vi "Periodic Tasks.vi"(0 "error in":errorcluster) -> ()   [LabVIEW 2019]
doc: "This VI runs in parallel to other tasks. It can contain as many user-defined periodic loops as you need. These can carry out PID or other sorts of timed response."
uses:
  dsinstructions.vi
  outputs.vi
  dsdata.vi
  constants.vi
  autoinfo.vi
  sensors.vi
  23a3f555-9381-40b3-b51f-cf650278d793.vi
  <vilib>/Rock Robotics/Network Tables/NT Write Number.vi
  8c2ce585-3354-44ed-b83e-22b56f2f092c.vi
  bb0a537a-131d-4120-96fe-e8b26fcd9fb4.vi
  <vilib>/Rock Robotics/Network Tables/NT Write String.vi
  70680724-1a9c-4240-8929-d59eeec2e4a0.vi
panel:
  out "Drive Sequencer":i32
  out "Subsystem Action":path
  out "Time Since Latch (ms)":u32
  out "Subsystem Sequencer":i32
  out "Drive Action":string
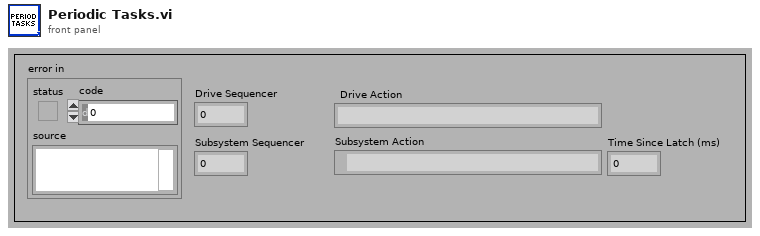
[diagram p1: front panel]
types:
  T1 = typedef "WPI_DriverStationRobotMode2.ctl" = enum16{"Autonomous Disabled", "Autonomous Enabled", "Teleop Disabled", "Teleop Enabled", "Disconnected", "Finish", "Test Disabled", "Test Enabled", "Emergency Stopped"}
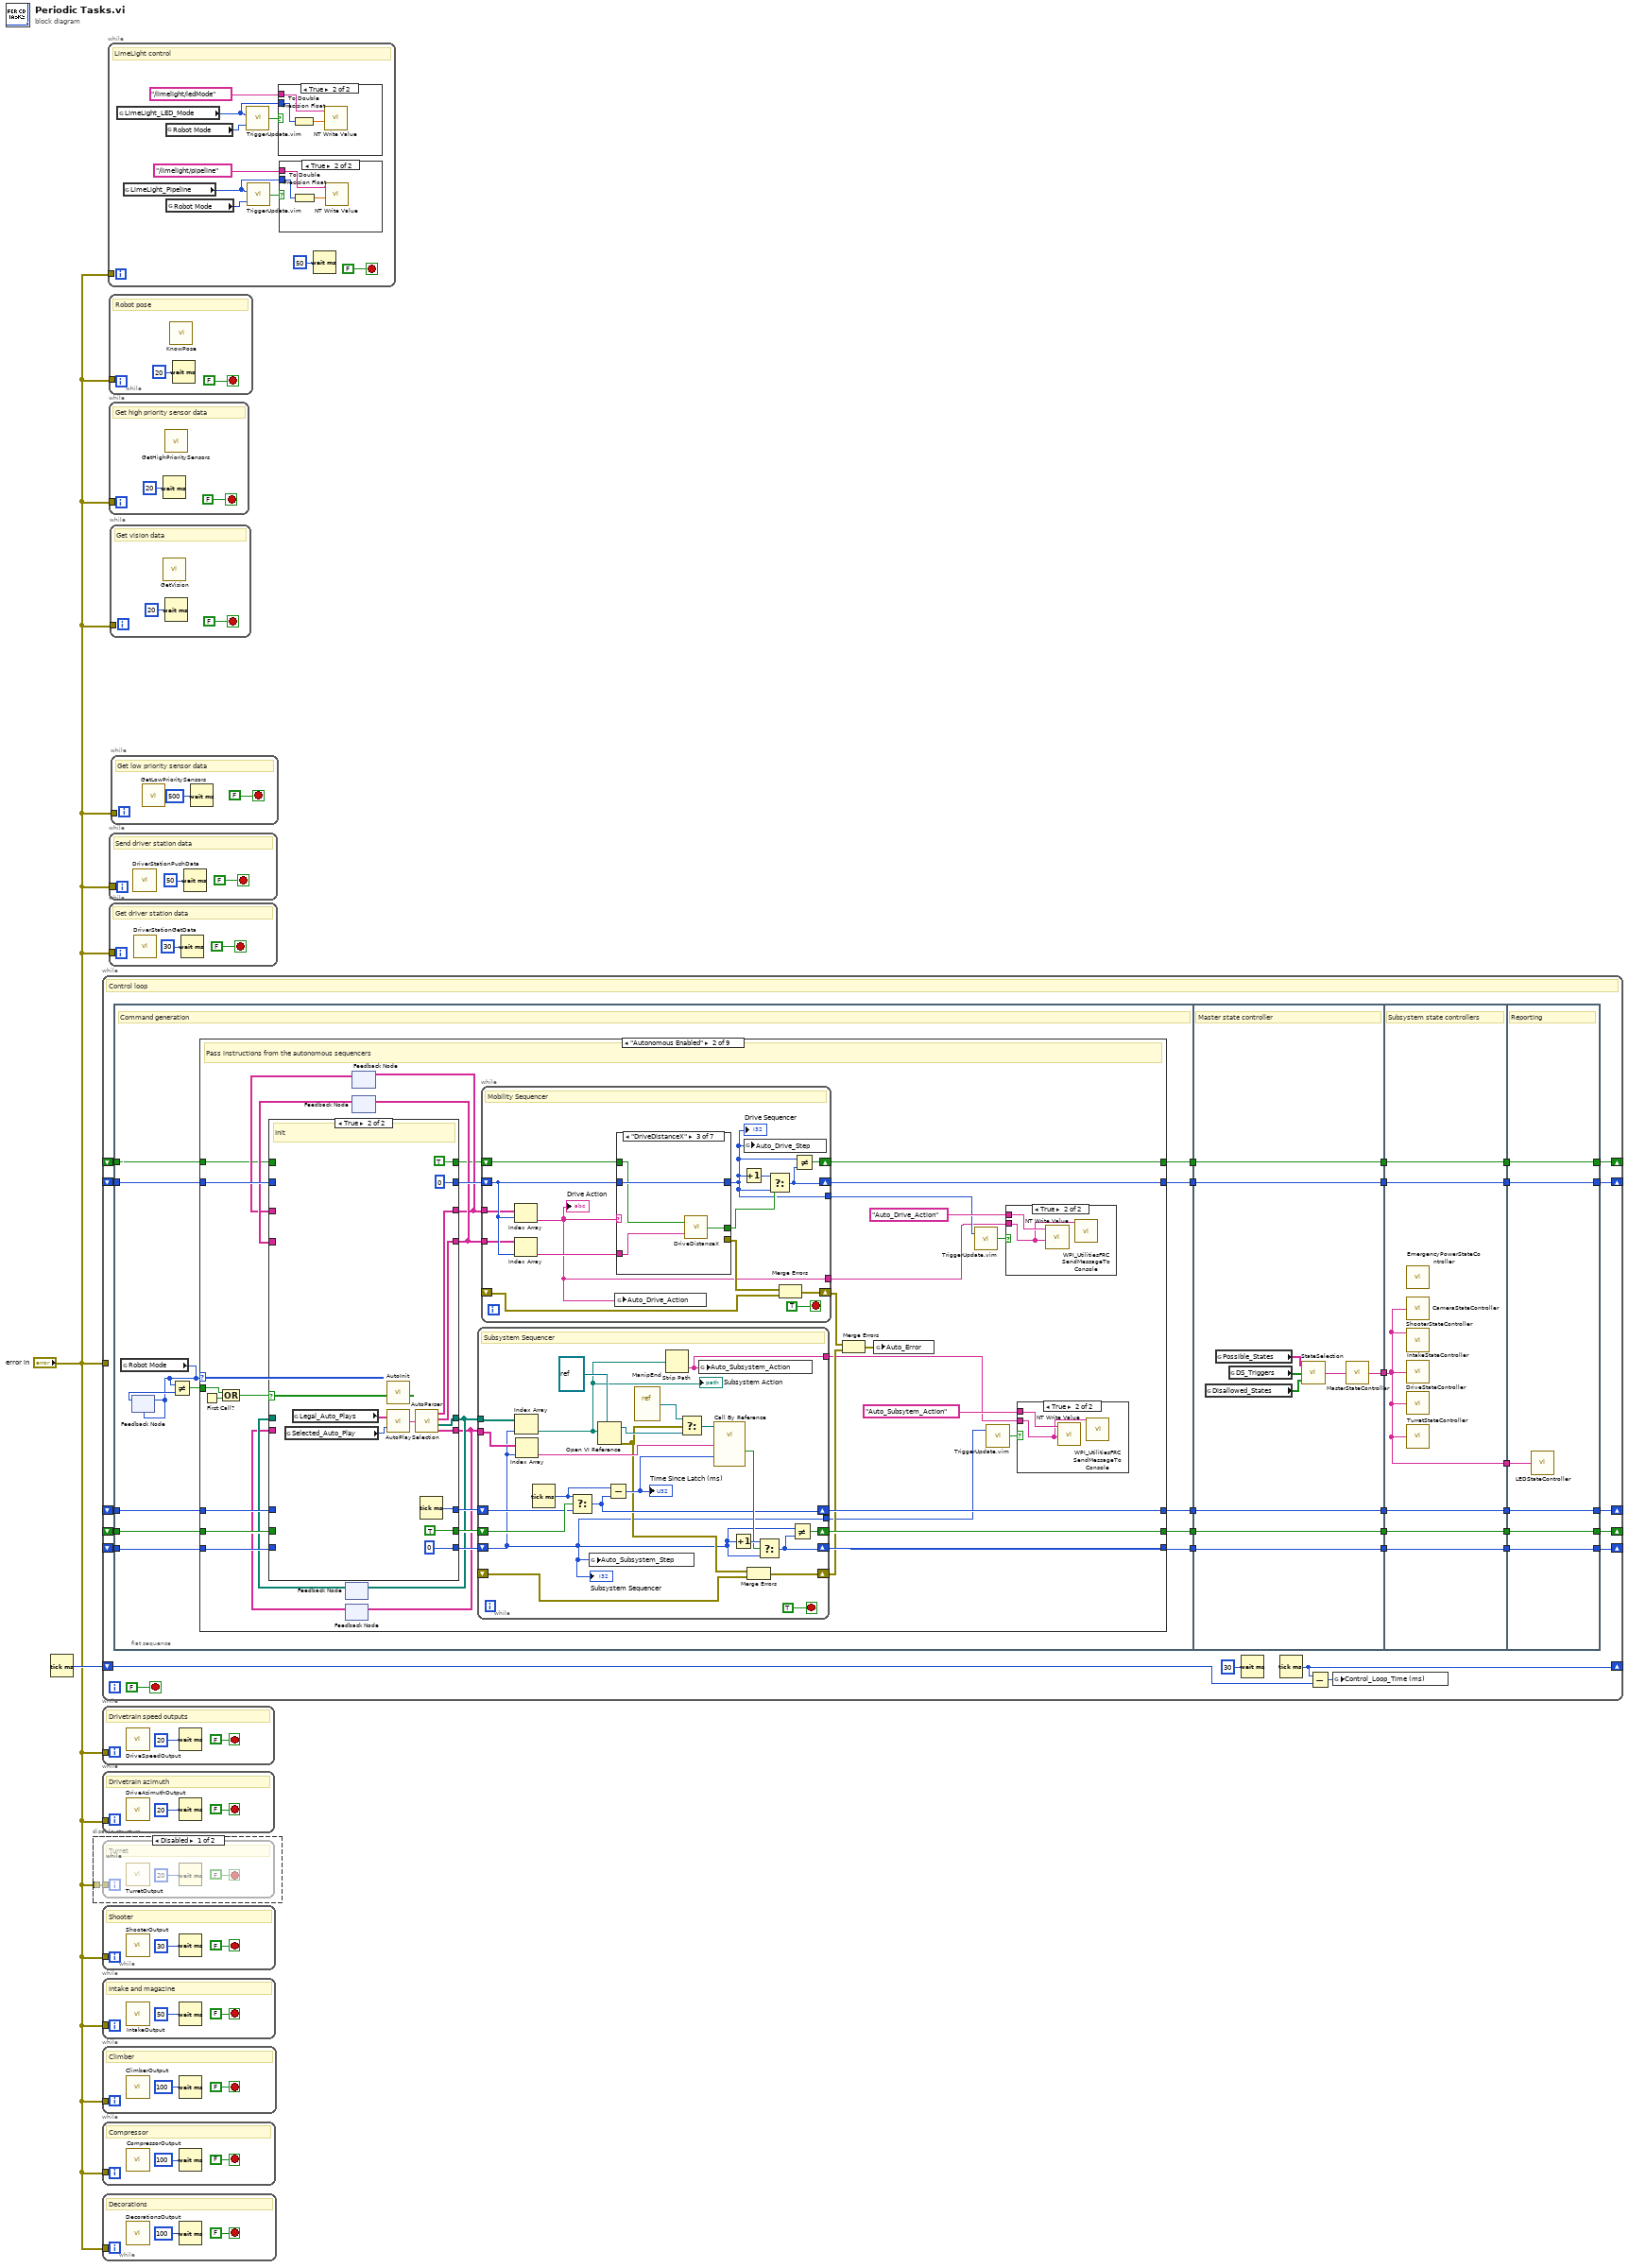
[diagram p0: block diagram]
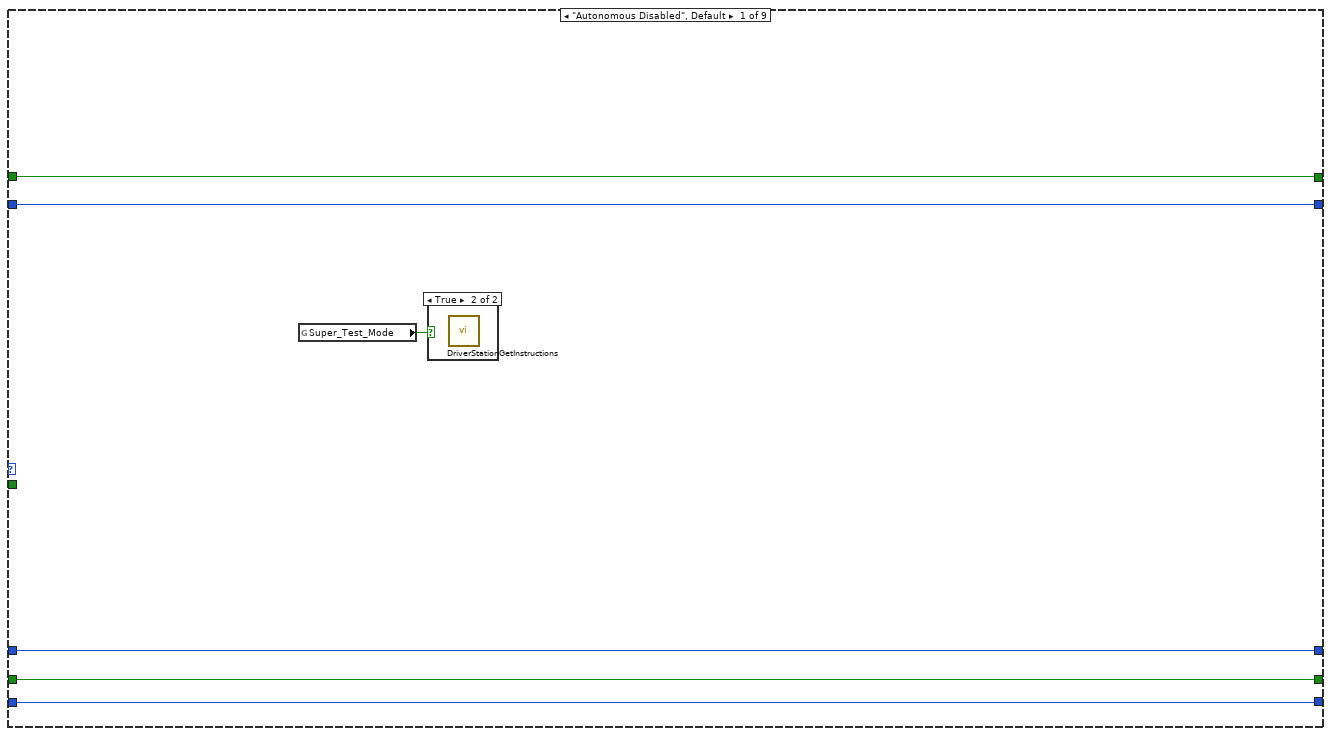
[diagram p5: hidden frame]
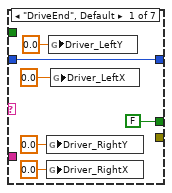
[diagram p9: hidden frame]
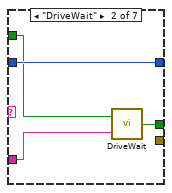
[diagram p10: hidden frame]
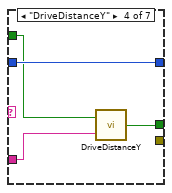
[diagram p11: hidden frame]
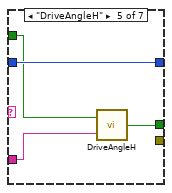
[diagram p12: hidden frame]
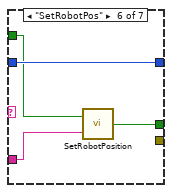
[diagram p13: hidden frame]
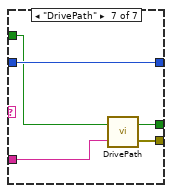
[diagram p14: hidden frame]
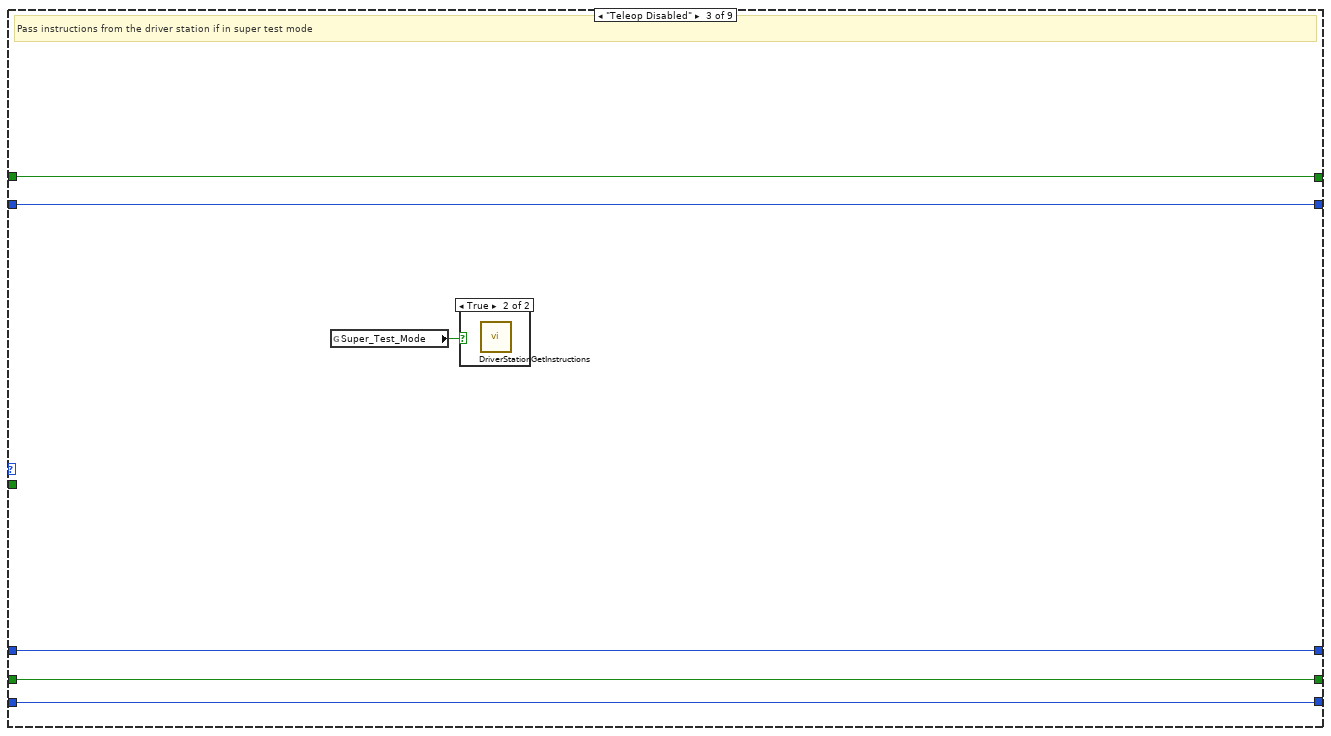
[diagram p16: hidden frame]
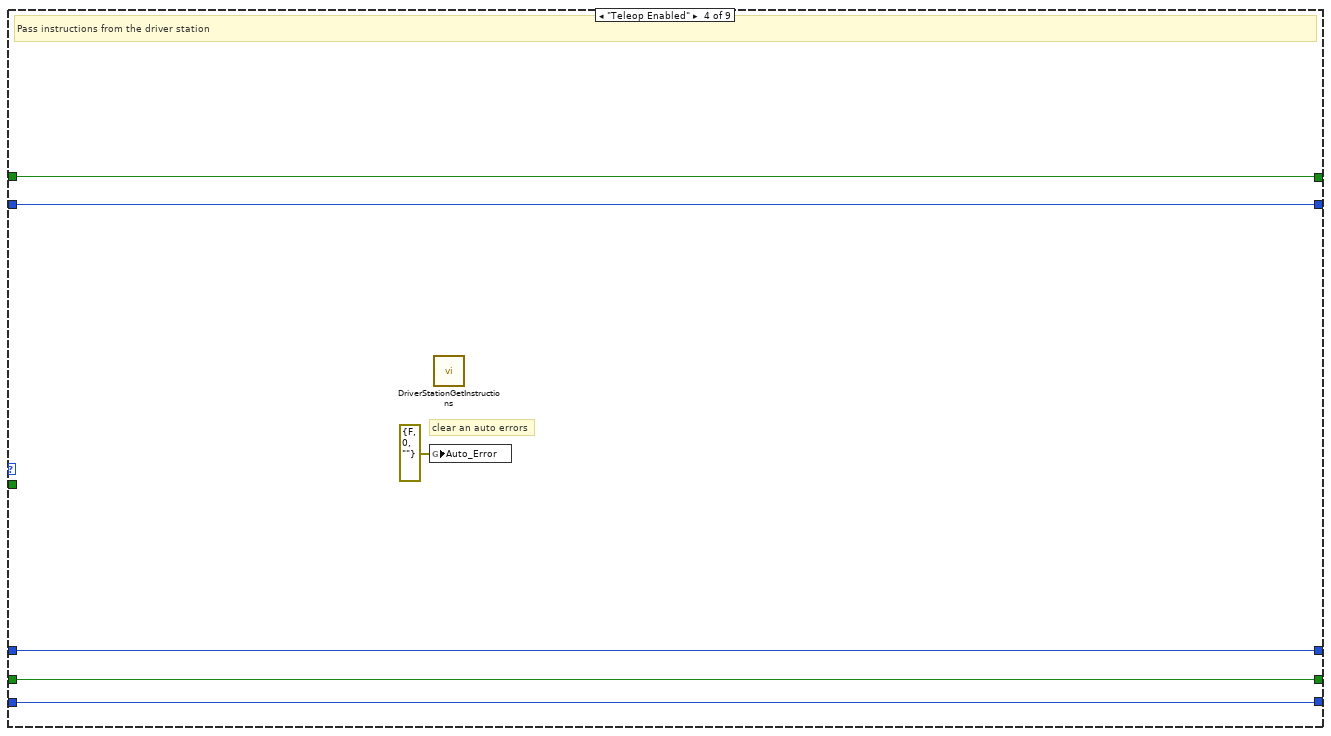
[diagram p18: hidden frame]
diagram:
  n1 = Tick Count (ms)() -> (millisecond timer value=w2:u32)
  n2 = disable-structure shown="Disabled" {
    disable-tunnel: "error in" -> [w3 _]
    frame Disabled {
      n3 = while {
        tunnel: w3 -> [_]
        stop <- FALSE stop-if-true
        # "Turret"
        n4 = call "TurretOutput.vi"() -> ()  [unwired: 1 in]
        n5 = Wait (ms)(milliseconds to wait=u32 20) -> ()  [unwired: 1 out]
      }
    }
    frame Enabled {
    }
  }
  n6 = while {
    tunnel: "error in" -> [_]
    shift-right: [w27] -> _
    shift-left: _ -> [w33]
    shift-right: [w28] -> _
    shift-left: _ -> [w34]
    shift-right: [w29] -> _
    shift-left: _ -> [w35]
    shift-right: [w25] -> _
    shift-left: _ -> [w24]
    shift-right: [w22] -> _
    shift-left: _ -> [w21]
    shift-right: [w20] -> _
    shift-left: w2 -> [w19]
    stop <- FALSE stop-if-true
    # "Control loop"
    n7 = flat-sequence {
      tunnel: w35 -> [w47]
      tunnel: w34 -> [w46]
      tunnel: w33 -> [w45]
      tunnel: [w50] -> w32
      tunnel: [w49] -> w31
      tunnel: [w48] -> w30
      tunnel: [w42] -> w26
      tunnel: w24 -> [w41]
      tunnel: [w40] -> w23
      tunnel: w21 -> [w39]
      tunnel: w32 -> [w234]
      tunnel: w31 -> [w233]
      tunnel: w30 -> [w232]
      tunnel: w26 -> [w231]
      tunnel: w23 -> [w230]
      tunnel: [w234] -> w17
      tunnel: [w233] -> w16
      tunnel: [w232] -> w15
      tunnel: [w231] -> w14
      tunnel: [w230] -> w13
      tunnel: [w225] -> w12
      tunnel: w17 -> [w240]
      tunnel: w16 -> [w239]
      tunnel: w15 -> [w238]
      tunnel: w14 -> [w237]
      tunnel: w13 -> [w236]
      tunnel: w12 -> [w235]
      tunnel: [w240] -> w11
      tunnel: [w239] -> w10
      tunnel: [w238] -> w9
      tunnel: [w237] -> w8
      tunnel: [w236] -> w7
      tunnel: [w235] -> w6
      tunnel: [w242] -> w22
      tunnel: [w243] -> w25
      tunnel: [w244] -> w27
      tunnel: [w245] -> w28
      tunnel: [w246] -> w29
      tunnel: w11 -> [w246]
      tunnel: w10 -> [w245]
      tunnel: w9 -> [w244]
      tunnel: w8 -> [w243]
      tunnel: w7 -> [w242]
      tunnel: w6 -> [w241]
      frame #0 {
        # "Command generation"
        n8 = global read "dsdata.vi" "Robot Mode"() -> (w38:T1)
        n9 = feedback-in #1(w38) -> ()
        n10 = feedback #1(w38) -> (w44:T1)
        n11 = Not Equal?(x=w38, y=w44) -> (x != y?=w43:bool)
        n12 = case shown="\"Autonomous Enabled\"" w38 {
          tunnel: w47 -> [w56 w90 w191 w197 w202 w207 w212 w217 w222]
          tunnel: w46 -> [w55 w88 w190 w196 w201 w206 w211 w216 w221]
          tunnel: w45 -> [w54 w87 w189 w195 w200 w205 w210 w215 w220]
          tunnel: [w56 w93 w191 w197 w202 w207 w212 w217 w222] -> w50
          tunnel: [w55 w92 w190 w196 w201 w206 w211 w216 w221] -> w49
          tunnel: [w54 w91 w189 w195 w200 w205 w210 w215 w220] -> w48
          tunnel: w43 -> [_ w82 _ _ _ _ _ _ _]
          tunnel: [w53 w76 w192 w198 w203 w208 w213 w218 w223] -> w42
          tunnel: w41 -> [w53 w75 w192 w198 w203 w208 w213 w218 w223]
          tunnel: [w52 w69 w193 w199 w204 w209 w214 w219 w224] -> w40
          tunnel: w39 -> [w52 w68 w193 w199 w204 w209 w214 w219 w224]
          frame "Autonomous Disabled", Default {
            n13 = global read "dsdata.vi" "Super_Test_Mode"() -> (w51:bool)
            n14 = case shown="True" w51 {
              frame False {
              }
              frame True {
                n15 = call "DriverStationGetInstructions.vi"() -> ()  [unwired: 12 in]
              }
            }
          }
          frame "Autonomous Enabled" {
            # "Pass instructions from the autonomous sequencers"
            n16 = First Call?() -> (First Call?: T/F=w83:bool)
            n17 = Compound Arithmetic op=OR(w82, w83) -> (w84:bool)
            n18 = feedback #2() -> (w79:path[])  [unwired: 1 in]
            n19 = feedback #3() -> (w78:string[])  [unwired: 1 in]
            n20 = feedback #4() -> (w71:string[])  [unwired: 1 in]
            n21 = feedback #5() -> (w72:string[])  [unwired: 1 in]
            n22 = case shown="True" w84 {
              tunnel: w87 -> [w150 _]
              tunnel: w88 -> [w151 _]
              tunnel: w90 -> [w152 _]
              tunnel: [w152 w164] -> w89
              tunnel: [w151 TRUE ("Advance Trigger")] -> w86
              tunnel: [w150 0] -> w85
              tunnel: [w149 w157] -> w81
              tunnel: [w148 w161] -> w80
              tunnel: w79 -> [w149 _]
              tunnel: w78 -> [w148 _]
              tunnel: [w147 0] -> w77
              tunnel: w75 -> [w147 _]
              tunnel: [w146 w159] -> w74
              tunnel: [w145 w158] -> w73
              tunnel: w72 -> [w146 _]
              tunnel: w71 -> [w145 _]
              tunnel: [w144 TRUE] -> w70
              tunnel: w68 -> [w144 _]
              frame False {
                # "Pass"
              }
              frame True {
                # "Init"
                n23 = global read "dsdata.vi" "Selected_Auto_Play"() -> (w155:u16)
                n24 = global read "constants.vi" "Legal_Auto_Plays"() -> (w154:string[])
                n25 = call "AutoInit.vi"() -> ()  [unwired: 1 in]
                n26 = call "AutoPlaySelection.vi"("Selected Auto Play"=w155, "Auto Plays"=w154) -> ("Autonomous Commands"=w153:string)
                n27 = call "AutoParser.vi"("Auto Play"=w153) -> ("Drive Mode Strings"=w158:string[], "Drive Command Strings"=w159:string[], "Subsystem VI References"=w157:path[], "Subsystem Command Strings"=w161:string[])
                n28 = Tick Count (ms)() -> (millisecond timer value=w164:u32)
              }
            }
            n29 = feedback-in #2(w81) -> ()
            n30 = feedback-in #3(w80) -> ()
            n31 = feedback-in #4(w73) -> ()
            n32 = feedback-in #5(w74) -> ()
            n33 = while {
              tunnel: w81 -> [w176]
              shift-right: [w183] -> w91
              shift-left: w85 -> [w165]
              shift-right: [w182] -> w92
              shift-left: w86 -> [w181]
              shift-right: [w179] -> w93
              shift-left: w89 -> [w180]
              tunnel: w80 -> [w175]
              shift-right: [w168] -> w66
              shift-left: _ -> [w167]
              tunnel: [w166] -> w58
              tunnel: [w165] -> w57
              stop <- TRUE stop-if-true
              # "Subsystem Sequencer"
              n34 = Index Array(array=w176, index=w165) -> (element=w170:path)
              "Subsystem Action" <- w170
              n35 = Index Array(array=w175, index=w165) -> (element=w174:string)
              n36 = Tick Count (ms)() -> (millisecond timer value=w178:u32)
              n37 = Select(t=w178, s=w181, f=w180) -> (s? t:f=w179:u32)
              n38 = global write "autoinfo.vi" "Auto_Subsystem_Step"(w165) -> ()
              n39 = Open VI Reference(type specifier VI Refnum (for type only)=refnum<vi> refnum, vi path=w170) -> (vi reference=w172:refnum<vi>, error out=w169:errorcluster)  [unwired: 4 in]
              n40 = Subtract(x=w178, y=w179) -> (x-y=w177:u32)
              "Time Since Latch (ms)" <- w177
              n41 = vi-ref "ManipEnd.vi"() -> (w171:refnum<vi>)
              n42 = Strip Path(path=w170) -> (name=w166:string)  [unwired: 1 out]
              n43 = Select(t=w171, s=w169, f=w172) -> (s? t:f=w173:refnum<vi>)
              n44 = global write "autoinfo.vi" "Auto_Subsystem_Action"(w166) -> ()
              n45 = call-by-ref "?"(reference=w173, "Time Since Latch"=w177, "Instruction String"=w174) -> ("Advance Trigger"=w184:bool)  [unwired: 1 in, 2 out]
              n46 = Increment(x=w165) -> (x+1=w186:i32)
              n47 = Merge Errors(w169, w167) -> (w168:errorcluster)
              n48 = Select(t=w186, s=w184, f=w165) -> (s? t:f=w183:i32)
              n49 = Not Equal?(x=w165, y=w183) -> (x != y?=w182:bool)
              "Subsystem Sequencer" <- w165
            }
            n50 = while {
              shift-right: [w106] -> w76
              shift-left: w77 -> [w110]
              tunnel: w73 -> [w109]
              tunnel: w74 -> [w108]
              shift-right: [w105] -> w69
              shift-left: w70 -> [w104]
              shift-right: [w102] -> w67
              shift-left: _ -> [w101]
              tunnel: [w99] -> w60
              tunnel: [w98] -> w59
              stop <- TRUE stop-if-true
              # "Mobility Sequencer"
              n51 = Index Array(array=w109, index=w110) -> (element=w98:string)
              "Drive Action" <- w98
              n52 = Index Array(array=w108, index=w110) -> (element=w107:string)
              n53 = global write "autoinfo.vi" "Auto_Drive_Action"(w98) -> ()
              n54 = case shown="\"DriveDistanceX\"" w98 {
                tunnel: w110 -> [w118 w122 w126 w130 w134 w138 w143]
                tunnel: [w118 w122 w126 w130 w134 w138 w143] -> w99
                tunnel: w107 -> [_ w119 w124 w127 w131 w136 w141]
                tunnel: [FALSE ("Increment") w121 w123 w129 w133 w137 w139] -> w100
                tunnel: w104 -> [_ w120 w125 w128 w132 w135 w142]
                tunnel: [_ _ _ _ _ _ w140] -> w103
                frame "DriveEnd", Default {
                  n55 = global write "dsinstructions.vi" "Driver_RightY"(0.0 ("Driver_RightX")) -> ()
                  n56 = global write "dsinstructions.vi" "Driver_RightX"(0.0 ("Driver_RightX")) -> ()
                  n57 = global write "dsinstructions.vi" "Driver_LeftY"(0.0 ("Driver_LeftY")) -> ()
                  n58 = global write "dsinstructions.vi" "Driver_LeftX"(0.0 ("Driver_RightX")) -> ()
                }
                frame "DriveWait" {
                  n59 = call "DriveWait.vi"("Parameter String"=w119, "Reinit"=w120) -> ("Increment"=w121:bool)
                }
                frame "DriveDistanceX" {
                  n60 = call "DriveDistanceX.vi"("Parameter String"=w124, "Reinit"=w125) -> ("Increment"=w123:bool)
                }
                frame "DriveDistanceY" {
                  n61 = call "DriveDistanceY.vi"("Parameter String"=w127, "Reinit"=w128) -> ("Increment"=w129:bool)
                }
                frame "DriveAngleH" {
                  n62 = call "DriveAngleH.vi"("Parameter String"=w131, "Reinit"=w132) -> ("Increment"=w133:bool)
                }
                frame "SetRobotPos" {
                  n63 = call "SetRobotPosition.vi"("Parameter String"=w136, "Reinit"=w135) -> ("Increment"=w137:bool)
                }
                frame "DrivePath" {
                  n64 = call "DrivePath.vi"("Parameter String"=w141, "Reinit"=w142) -> ("Path Follow Error"=w140:errorcluster, "Increment"=w139:bool)
                }
              }
              "Drive Sequencer" <- w99
              n65 = Increment(x=w99) -> (x+1=w111:i32)
              n66 = global write "autoinfo.vi" "Auto_Drive_Step"(w99) -> ()
              n67 = Select(t=w111, s=w100, f=w99) -> (s? t:f=w106:i32)
              n68 = Merge Errors(w103, w101) -> (w102:errorcluster)
              n69 = Not Equal?(x=w99, y=w106) -> (x != y?=w105:bool)
            }
            n70 = Merge Errors(w67, w66) -> (w65:errorcluster)
            n71 = global write "autoinfo.vi" "Auto_Error"(w65) -> ()
            n72 = call "TriggerUpdate.vim"("Trigger"=w60) -> ("Update"=w64:bool)  [unwired: 1 in]
            n73 = call "TriggerUpdate.vim"("Trigger"=w57) -> ("Update"=w62:bool)  [unwired: 1 in]
            n74 = case shown="True" w64 {
              tunnel: w59 -> [_ w96]
              tunnel: "Auto_Drive_Action" ("Name") -> [_ w97]
              frame False {
              }
              frame True {
                n75 = call-poly <vilib>:"NT Write Value.vi"("String"=w96, "Name"=w97) -> ()  [unwired: 9 in, 1 out]
                n76 = call <vilib>:"WPI_UtilitiesFRC SendMessageToConsole.vi"("Message"=w96) -> ()  [unwired: 14 in, 1 out]
              }
            }
            n77 = case shown="True" w62 {
              tunnel: w58 -> [_ w94]
              tunnel: "Auto_Subsytem_Action" ("Name") -> [_ w95]
              frame False {
              }
              frame True {
                n78 = call-poly <vilib>:"NT Write Value.vi"("String"=w94, "Name"=w95) -> ()  [unwired: 9 in, 1 out]
                n79 = call <vilib>:"WPI_UtilitiesFRC SendMessageToConsole.vi"("Message"=w94) -> ()  [unwired: 14 in, 1 out]
              }
            }
          }
          frame "Teleop Disabled" {
            # "Pass instructions from the driver station if in super test mode"
            n80 = global read "dsdata.vi" "Super_Test_Mode"() -> (w188:bool)
            n81 = case shown="True" w188 {
              frame False {
              }
              frame True {
                n82 = call "DriverStationGetInstructions.vi"() -> ()  [unwired: 12 in]
              }
            }
          }
          frame "Teleop Enabled" {
            # "clear an auto errors"
            # "Pass instructions from the driver station"
            n83 = global write "autoinfo.vi" "Auto_Error"(errorcluster {"status"=FALSE, "code"=0, "source"=""} ("Auto_Error")) -> ()
            n84 = call "DriverStationGetInstructions.vi"() -> ()  [unwired: 12 in]
          }
          frame "Finish" {
            # "Clean up operations are in the Finish.vi in RobotMain.vi"
          }
          frame "Test Disabled" {
            # "We are not using the testing mode"
          }
          frame "Test Enabled" {
            # "We are not using the testing mode"
          }
          frame "Disconnected" {
          }
          frame "Emergency Stopped" {
          }
        }
      }
      frame #1 {
        # "Master state controller"
        n85 = global read "constants.vi" "Disallowed_States"() -> (w227:bool[])
        n86 = global read "constants.vi" "Possible_States"() -> (w228:string[])
        n87 = global read "dsinstructions.vi" "DS_Triggers"() -> (w229:bool[])
        n88 = call "StateSelection.vi"("Disallowed States"=w227, "State Triggers"=w229, "State Names"=w228) -> ("Selected State"=w226:string)
        n89 = call "MasterStateController.vi"("Selected State (In)"=w226) -> ("Selected State (Out)"=w225:string)
      }
      frame #2 {
        # "Subsystem state controllers"
        n90 = call "EmergencyPowerStateController.vi"() -> ()  [unwired: 1 in]
        n91 = call "CameraStateController.vi"("Selected State (In)"=w235) -> ()  [unwired: 1 out]
        n92 = call "ShooterStateController.vi"("Selected State (In)"=w235) -> ()  [unwired: 3 in, 1 out]
        n93 = call "IntakeStateController.vi"("Selected State (In)"=w235) -> ()  [unwired: 1 out]
        n94 = call "DriveStateController.vi"("Selected State (In)"=w235) -> ()  [unwired: 1 out]
        n95 = call "TurretStateController.vi"("Selected State (In)"=w235) -> ()  [unwired: 1 out]
      }
      frame #3 {
        # "Reporting"
        n96 = call "LEDStateController.vi"("Selected State (In)"=w241) -> ()  [unwired: 1 out]
      }
    }
    n97 = Wait (ms)(milliseconds to wait=u32 30) -> ()  [unwired: 1 out]
    n98 = Tick Count (ms)() -> (millisecond timer value=w20:u32)
    n99 = Subtract(x=w20, y=w19) -> (x-y=w18:u32)
    n100 = global write "sensors.vi" "Control_Loop_Time (ms)"(w18) -> ()
  }
  n101 = while {
    tunnel: "error in" -> [_]
    stop <- FALSE stop-if-true
    # "Drivetrain speed outputs"
    n102 = call "DriveSpeedOutput.vi"() -> ()  [unwired: 1 in]
    n103 = Wait (ms)(milliseconds to wait=u32 20) -> ()  [unwired: 1 out]
  }
  n104 = while {
    tunnel: "error in" -> [_]
    stop <- FALSE stop-if-true
    # "Drivetrain azimuth"
    n105 = call "DriveAzimuthOutput.vi"() -> ()  [unwired: 1 in]
    n106 = Wait (ms)(milliseconds to wait=u32 20) -> ()  [unwired: 1 out]
  }
  n107 = while {
    tunnel: "error in" -> [_]
    stop <- FALSE stop-if-true
    # "Shooter"
    n108 = call "ShooterOutput.vi"() -> ()  [unwired: 1 in]
    n109 = Wait (ms)(milliseconds to wait=u32 30) -> ()  [unwired: 1 out]
  }
  n110 = while {
    tunnel: "error in" -> [_]
    stop <- FALSE stop-if-true
    # "Intake and magazine"
    n111 = call "IntakeOutput.vi"() -> ()  [unwired: 1 in]
    n112 = Wait (ms)(milliseconds to wait=u32 50) -> ()  [unwired: 1 out]
  }
  n113 = while {
    tunnel: "error in" -> [_]
    stop <- FALSE stop-if-true
    # "Climber"
    n114 = call "ClimberOutput.vi"() -> ()  [unwired: 1 in]
    n115 = Wait (ms)(milliseconds to wait=u32 100) -> ()  [unwired: 1 out]
  }
  n116 = while {
    tunnel: "error in" -> [_]
    stop <- FALSE stop-if-true
    # "Compressor"
    n117 = call "CompressorOutput.vi"() -> ()  [unwired: 1 in]
    n118 = Wait (ms)(milliseconds to wait=u32 100) -> ()  [unwired: 1 out]
  }
  n119 = while {
    tunnel: "error in" -> [_]
    stop <- FALSE stop-if-true
    # "Decorations"
    n120 = call "DecorationsOutput.vi"() -> ()  [unwired: 1 in]
    n121 = Wait (ms)(milliseconds to wait=u32 100) -> ()  [unwired: 1 out]
  }
  n122 = while {
    tunnel: "error in" -> [_]
    stop <- FALSE stop-if-true
    # "LimeLight control"
    n123 = global read "outputs.vi" "LimeLight_LED_Mode"() -> (w261:i64)
    n124 = global read "outputs.vi" "LimeLight_Pipeline"() -> (w267:i64)
    n125 = global read "dsdata.vi" "Robot Mode"() -> (w263:T1)
    n126 = global read "dsdata.vi" "Robot Mode"() -> (w269:T1)
    n127 = call "TriggerUpdate.vim"("Robot Mode"=w263, "Trigger"=w261) -> ("Update"=w264:bool)
    n128 = call "TriggerUpdate.vim"("Robot Mode"=w269, "Trigger"=w267) -> ("Update"=w270:bool)
    n129 = case shown="True" w264 {
      tunnel: w261 -> [_ w273]
      tunnel: "/limelight/ledMode" ("Name") -> [_ w272]
      frame False {
      }
      frame True {
        n130 = To Double Precision Float(number=w273) -> (double precision float=w271:dbl)
        n131 = call-poly <vilib>:"NT Write Value.vi"("Numeric"=w271, "Name"=w272) -> ()  [unwired: 9 in, 1 out]
      }
    }
    n132 = case shown="True" w270 {
      tunnel: w267 -> [_ w276]
      tunnel: "/limelight/pipeline" ("Name") -> [_ w275]
      frame False {
      }
      frame True {
        n133 = To Double Precision Float(number=w276) -> (double precision float=w274:dbl)
        n134 = call-poly <vilib>:"NT Write Value.vi"("Numeric"=w274, "Name"=w275) -> ()  [unwired: 9 in, 1 out]
      }
    }
    n135 = Wait (ms)(milliseconds to wait=u32 50) -> ()  [unwired: 1 out]
  }
  n136 = while {
    tunnel: "error in" -> [_]
    stop <- FALSE stop-if-true
    # "Robot pose"
    n137 = call "KnowPose.vi"() -> ()  [unwired: 1 in]
    n138 = Wait (ms)(milliseconds to wait=u32 20) -> ()  [unwired: 1 out]
  }
  n139 = while {
    tunnel: "error in" -> [_]
    stop <- FALSE stop-if-true
    # "Get high priority sensor data"
    n140 = Wait (ms)(milliseconds to wait=u32 20) -> ()  [unwired: 1 out]
    n141 = call "GetHighPrioritySensors.vi"() -> ()  [unwired: 1 in]
  }
  n142 = while {
    tunnel: "error in" -> [_]
    stop <- FALSE stop-if-true
    # "Get driver station data"
    n143 = call "DriverStationGetData.vi"() -> ()  [unwired: 1 in]
    n144 = Wait (ms)(milliseconds to wait=u32 30) -> ()  [unwired: 1 out]
  }
  n145 = while {
    tunnel: "error in" -> [_]
    stop <- FALSE stop-if-true
    # "Send driver station data"
    n146 = call "DriverStationPushData.vi"() -> ()  [unwired: 12 in]
    n147 = Wait (ms)(milliseconds to wait=u32 50) -> ()  [unwired: 1 out]
  }
  n148 = while {
    tunnel: "error in" -> [_]
    stop <- FALSE stop-if-true
    # "Get vision data"
    n149 = call "GetVision.vi"() -> ()  [unwired: 12 in]
    n150 = Wait (ms)(milliseconds to wait=u32 20) -> ()  [unwired: 1 out]
  }
  n151 = while {
    tunnel: "error in" -> [_]
    stop <- FALSE stop-if-true
    # "Get low priority sensor data"
    n152 = call "GetLowPrioritySensors.vi"() -> ()  [unwired: 12 in]
    n153 = Wait (ms)(milliseconds to wait=u32 500) -> ()  [unwired: 1 out]
  }
